vi "Format Date Time String part 5.vi"() -> ()   [LabVIEW 2020]
panel:
  out "date/time string":string
  in  "time stamp":timestamp format="%<%I:%M %p\n%x>T"
  in  "time format string (%c)":string
  # "Part 5"
  # "Format Date/Time String"
  # "Format Code Value \n<%a> abbreviated weekday name (for example Wed) \n<%A> full weekday name (for example Wednesday) \n<%b> abbreviated month name (for example Jun) \n<%B> full month name (for example June) \n<%c> locale-specific default date and time \n<%d> day of month (01–31) \n<%H> hour (24-hour clock) (00–23) \n<%I> hour (12-hour clock) (01–12) \n<%j> day number of the year (001–366) \n<%m> month number (01–12) \n<%M> minute (00–59) \n<%p> AM or PM flag \n<%S> second (00–59)"
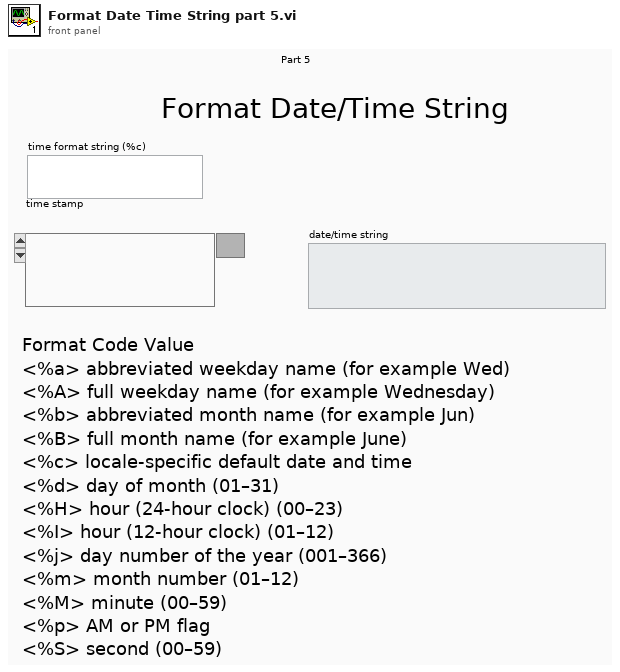
[diagram p1: front panel]
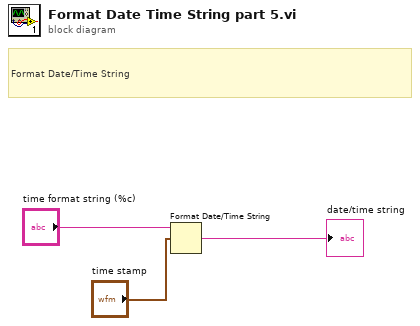
[diagram p0: block diagram]
diagram:
  # "Format Date/Time String"
  n1 = Format Date/Time String(time format string (%c)="time format string (%c)", seconds (now)="time stamp") -> (date/time string=→"date/time string":string)  [unwired: 1 in]
